vi "Config Data.vi"() -> ()   [LabVIEW 2014]
panel:
  in  "Config Data":cluster{"DriveTrainLogFile":path}
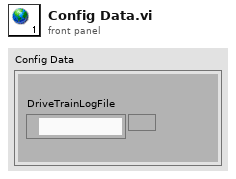
[diagram p1: front panel]
diagram:
